vi "driveShifterControl.vi"   [LabVIEW 2018]
uses:
  driveShiftEnum.ctl
  <vilib>/Rock Robotics/WPI/Utilities/WPI_GetSetVariantRefNum.vi
types:
  T1 = typedef "WPI_JoystickDevRef.ctl" = cluster{"Device":T2}
  T2 = typedef "WPI_JoystickDeviceEnum.ctl" = enum16{"USB 0", "USB 1", "USB 2", "USB 3", "USB 4", "USB 5"}
  T3 = typedef "driveShiftEnum.ctl" = enum16{"Low", "High"}
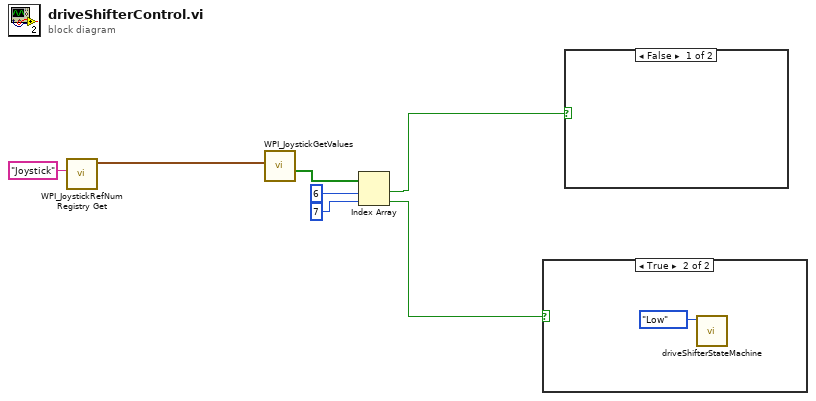
[diagram p0: block diagram]
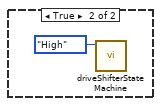
[diagram p3: hidden frame]
diagram:
  n1 = call <vilib>:"WPI_JoystickRefNum Registry Get.vi"("refnum name"="Joystick") -> ("JoystickDevRef"=w6:T1)  [unwired: 9 in, 1 out]
  n2 = call <vilib>:"WPI_JoystickGetValues.vi"("JoystickDevRef"=w6) -> ("Buttons"=w5:bool[])  [unwired: 6 in, 4 out]
  n3 = Index Array(array=w5, index #1=6 ("index"), index #2=7 ("index")) -> (element #1=w2:bool, element #2=w1:bool)
  n4 = case shown="True" w1 {
    frame False {
    }
    frame True {
      n5 = call "driveShifterStateMachine.vi"("Drive Shift State"=driveShiftEnum."Low") -> ()  [unwired: 11 in]
    }
  }
  n6 = case shown="False" w2 {
    frame False {
    }
    frame True {
      n7 = call "driveShifterStateMachine.vi"("Drive Shift State"=driveShiftEnum."High") -> ()  [unwired: 11 in]
    }
  }
